vi "Begin.vi"(8 "error in":errorcluster) -> (0 "error out":errorcluster)   [LabVIEW 2017]
doc: "Called before other user functions, this VI is expected to open initial I/O refnums, load in file data, and do all program initialization. Notice that the <B>error out</B> terminal is simply used for data flow. Wiring it to other structures or subVIs ensures that this VI runs first."
uses:
  <vilib>/Rock Robotics/WPI/DriverStation/WPI_DriverStationRobotMode2.ctl
  <vilib>/Rock Robotics/WPI/Solenoid/WPI_SolenoidValue.ctl
  Globals/Robot Global Data.vi
  <vilib>/Rock Robotics/Network Tables/NT Write String Array.vi
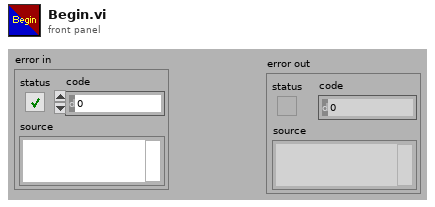
[diagram p1: front panel]
types:
  T1 = typedef "WPI_SolenoidValue.ctl" = enum16{"Off", "On", "Forward", "Reverse"}
  T2 = typedef "WPI_DriverStationRobotMode2.ctl" = enum16{"Autonomous Disabled", "Autonomous Enabled", "Teleop Disabled", "Teleop Enabled", "Disconnected", "Finish", "Test Disabled", "Test Enabled", "Emergency Stopped"}
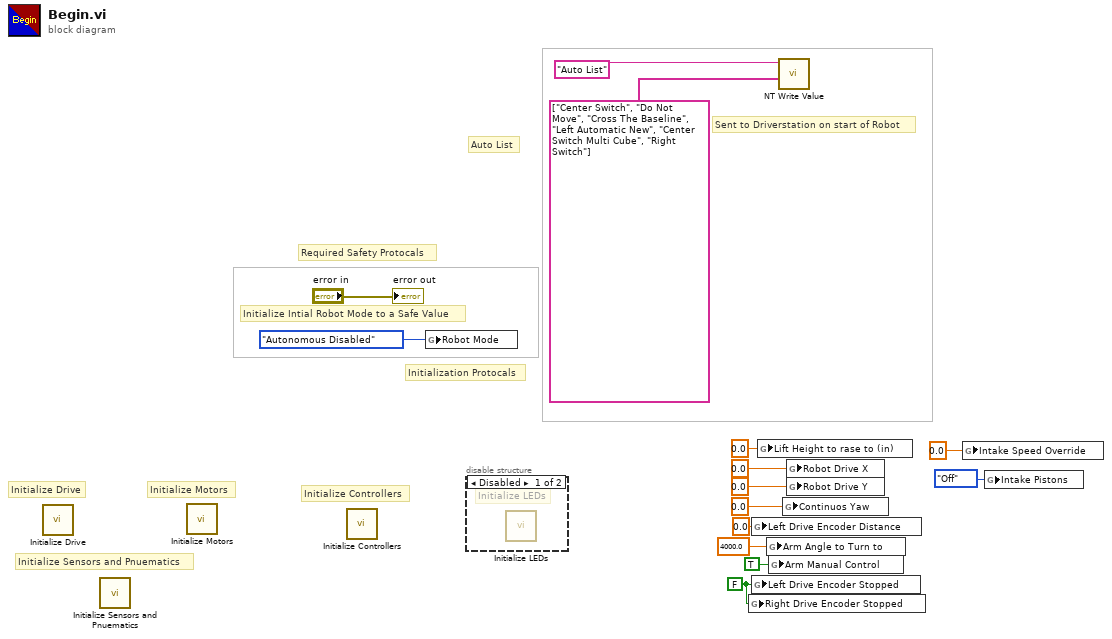
[diagram p0: block diagram]
diagram:
  w2 = FALSE ("Left Drive Encoder Stopped")
  # "Initialize Controllers"
  # "Initialize Sensors and Pnuematics"
  # "Initialize Motors"
  # "Initialize Drive"
  # "Initialization Protocals"
  # "Required Safety Protocals"
  # "Initialize Intial Robot Mode to a Safe Value"
  # "Sent to Driverstation on start of Robot"
  # "Auto List"
  n1 = call "Initialize Drive.vi"() -> ()  [unwired: 12 in]
  n2 = call "Initialize Sensors and Pnuematics.vi"() -> ()  [unwired: 12 in]
  n3 = call "Initialize Motors.vi"() -> ()  [unwired: 12 in]
  n4 = call "Initialize Controllers.vi"() -> ()  [unwired: 12 in]
  n5 = global write "Robot Global Data.vi" "Robot Mode"(WPI_DriverStationRobotMode2."Autonomous Disabled" ("Robot Mode")) -> ()
  n6 = disable-structure shown="Disabled" {
    frame Disabled {
      # "Initialize LEDs"
      n7 = call "Initialize LEDs.vi"() -> ()  [unwired: 12 in]
    }
    frame Enabled {
    }
  }
  n8 = global write "Robot Global Data.vi" "Right Drive Encoder Stopped"(w2) -> ()
  n9 = global write "Robot Global Data.vi" "Left Drive Encoder Distance"(0.0 ("Lift Height to rase to (in)")) -> ()
  n10 = global write "Robot Global Data.vi" "Left Drive Encoder Stopped"(w2) -> ()
  n11 = global write "Robot Global Data.vi" "Lift Height to rase to (in)"(0.0 ("Lift Height to rase to (in)")) -> ()
  n12 = global write "Robot Global Data.vi" "Arm Angle to Turn to"(4000.0 ("Lift Height to rase to (in)")) -> ()
  n13 = global write "Robot Global Data.vi" "Arm Manual Control"(TRUE ("Arm Manual Control")) -> ()
  n14 = call-poly <vilib>:"NT Write Value.vi"("String Array"=string[] ["Center Switch", "Do Not Move", "Cross The Baseline", "Left Automatic New", "Center Switch Multi Cube", "Right Switch"], "Name"="Auto List") -> ()  [unwired: 9 in, 1 out]
  n15 = global write "Robot Global Data.vi" "Continuos Yaw"(0.0 ("Lift Height to rase to (in)")) -> ()
  n16 = global write "Robot Global Data.vi" "Robot Drive X"(0.0 ("Lift Height to rase to (in)")) -> ()
  n17 = global write "Robot Global Data.vi" "Robot Drive Y"(0.0 ("Lift Height to rase to (in)")) -> ()
  n18 = global write "Robot Global Data.vi" "Intake Speed Override"(0.0 ("Lift Height to rase to (in)")) -> ()
  n19 = global write "Robot Global Data.vi" "Intake Pistons"(WPI_SolenoidValue."Off" ("Intake Pistons")) -> ()
  "error out" <- "error in"
